vi "Main.vi"() -> ()   [LabVIEW 2018]
uses:
  G .NET.lvlib
panel:
  out "Array Size":i32
  out ".NET Type Name":string
  out "HTTP Request Messages Out":T1(array[cluster]) {"Request Line"."Method" items=["GET", "HEAD", "POST", "PUT", "DELETE", "CONNECT", "OPTIONS"]}
  in  "HTTP Request Messages In":T1(array[cluster])=[{"Request Line"={"Method"=0, "URI"="/images/cats.html", "Protocol"="HTTP/1.1"}, "Header Fields"={"Host"="www.animals.com", "Accept"="image/gif image/jpeg", "Accept-Language"="en-GB", "Accept-Encoding"="gzip, deflate", "User-Agent"="Mozilla/5.0"}}, {"Request Line"={"Method"=0, "URI"="/pages/dogs.html", "Protocol"="HTTP/1.1"}, "Header Fields"={"Host"="www.animals.com", "Accept"="*/*", "Accept-Language"="en-US,en;q=0.9", "Accept-Encoding"="gzip, deflate", "User-Agent"="Chrome/100.0.4896.60"}}, {"Request Line"={"Method"=0, "URI"="/Identity/Dropdown?n=...", "Protocol"="HTTP/1.1"}, "Header Fields"={"Host"="www.bing.com", "Accept"="text/html text/plain image/gif image/jpeg", "Accept-Language"="en-US,en;q=0.9", "Accept-Encoding"="gzip, deflate, br", "User-Agent"="Edg/100.0.1185.29"}}] {"Request Line"."Method" items=["GET", "HEAD", "POST", "PUT", "DELETE", "CONNECT", "OPTIONS"]}
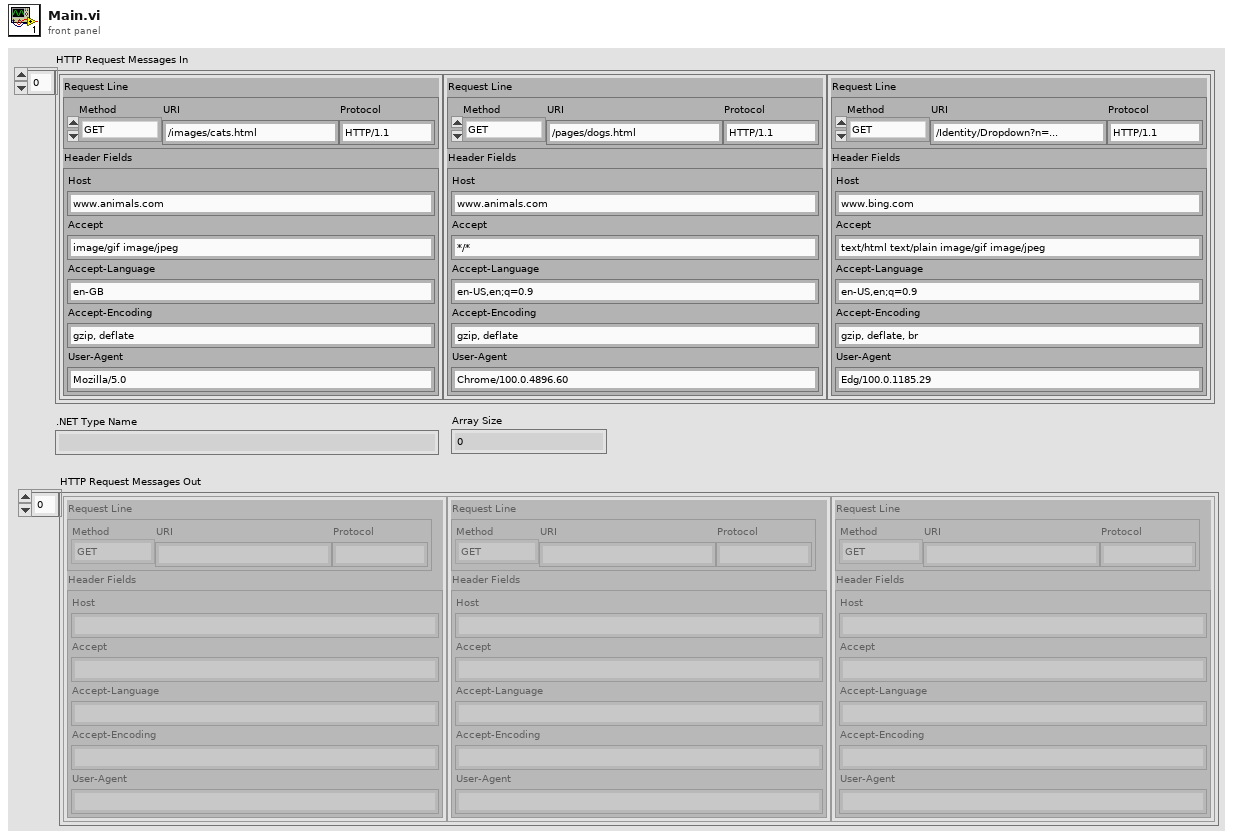
[diagram p1: front panel]
types:
  T1 = cluster{"Request Line":cluster{"Method":u16, "URI":string, "Protocol":string}, "Header Fields":cluster{"Host":string, "Accept":string, "Accept-Language":string, "Accept-Encoding":string, "User-Agent":string}}[]
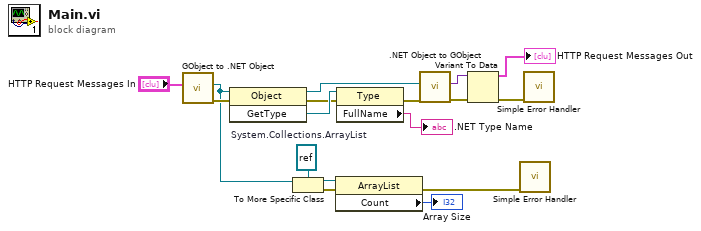
[diagram p0: block diagram]
diagram:
  w6 = refnum<k24> refnum  # System.Collections.ArrayList
  n1 = call "GObject to .NET Object.vi"("G Object"="HTTP Request Messages In") -> ("error out"=w12:errorcluster, ".NET Object"=w3:refnum<k24>)  [unwired: 9 in]
  n2 = invoke class="Object" method="GetType"(reference=w3, error in=w12) -> (reference out=w9:refnum<k24>, error out=w10:errorcluster, "GetType"=w11:refnum<k24>)  [unwired: 1 in]
  n3 = To More Specific Class(target class=w6, reference=w3) -> (specific class reference=w4:refnum<k24>, error out=w5:errorcluster)  [unwired: 1 in]
  n4 = property class="ArrayList"(reference=w4, error in=w5) -> (error out=w1:errorcluster, "Count"=→"Array Size":i32)  [unwired: 1 out]
  n5 = property class="Type"(reference=w11, error in=w10) -> (error out=w8:errorcluster, "FullName"=→".NET Type Name":string)  [unwired: 1 out]
  n6 = call ".NET Object to GObject.vi"("error in (no error)"=w8, ".NET Object"=w9) -> ("error out"=w17:errorcluster, "G Object"=w16:variant)  [unwired: 8 in]
  n7 = Variant To Data(error in=w17, Variant=w16) -> (data=→"HTTP Request Messages Out":T1, error out=w15:errorcluster)  [unwired: 1 in]
  n8 = call <vilib>:"Simple Error Handler.vi"("error in (no error)"=w1) -> ()  [unwired: 4 in, 5 out]
  n9 = call <vilib>:"Simple Error Handler.vi"("error in (no error)"=w15) -> ()  [unwired: 4 in, 5 out]
